vi "Write Data.vi"(8 "error in (no error)":errorcluster, 10 "Data":variant, 11 "Update Settings in":refnum<class "Update Settings.lvclass">) -> (0 "error out":errorcluster, 3 "Update Settings out":refnum<class "Update Settings.lvclass">)   [LabVIEW 2014, in "Update Settings.lvclass"]
uses:
  Update Settings.lvclass
  Update Settings.lvclass/Update Settings.ctl
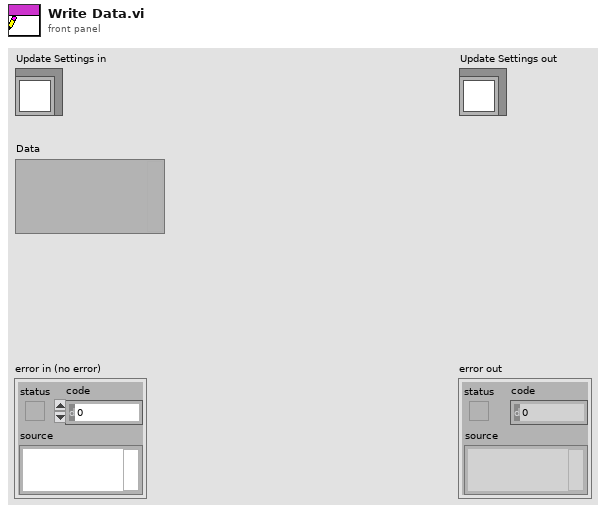
[diagram p1: front panel]
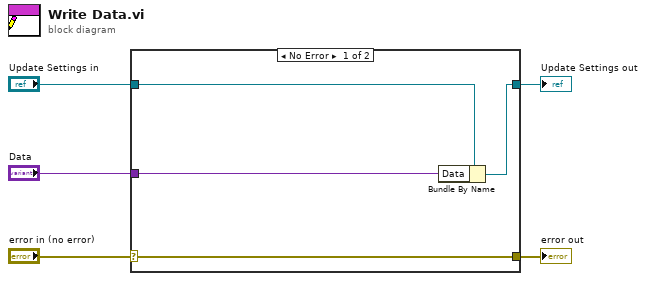
[diagram p0: block diagram]
diagram:
  n1 = case shown="No Error" "error in (no error)" {
    selector: "error in (no error)" -> [w9 w10]
    tunnel: [w9 w10] -> w4
    tunnel: [w7 w11] -> w2
    tunnel: "Update Settings in" -> [w8 w11]
    tunnel: "Data" -> [w6 _]
    frame No Error {
      n2 = Bundle By Name(cluster=w8, "Data"=w6) -> (w7:refnum<class "Update Settings.lvclass">)
    }
    frame Error {
    }
  }
  "error out" <- w4
  "Update Settings out" <- w2
